vi "Export Configuration.vi"(8 "error in":errorcluster, 10 "configuration file path":path, 11 "data sharing framework custom device":T1 format="%.0x") -> (0 "error out":errorcluster, 2 "actual configuration file path":path, 3 "data sharing framework custom device":T1 format="%.0x")   [LabVIEW 2017, in "Data Sharing Framework Custom Device Scripting.lvlib"]
doc: "Creates or updates a Data Sharing Framework configuration file (.dsf) based on the custom device configuration in the system definition file."
uses:
  Data Sharing Framework Custom Device Scripting.lvlib
  <vilib>/NI Veristand/Custom Device API/Custom Device Item Ref.ctl
  Shared/DSF Shared.lvlib
  System Explorer/DSF System Explorer.lvlib
  DSF Core.lvlibp/Classes/Configuration Session/Configuration Session.lvclass
  <vilib>/NI VeriStand/Custom Device API/Custom Device API.lvlib
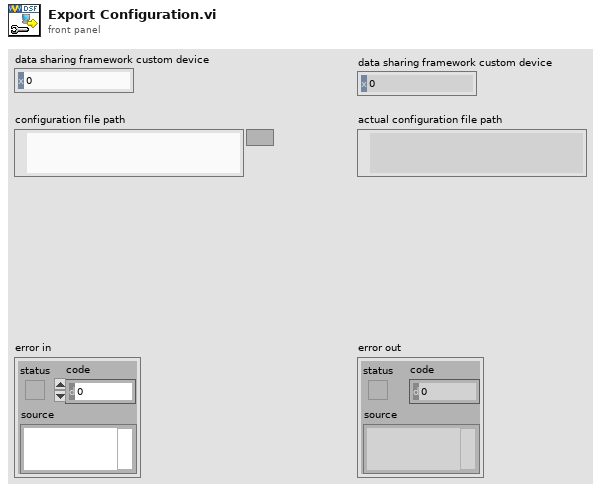
[diagram p1: front panel]
types:
  T1 = typedef "Custom Device API.lvlib/Custom Device Item Ref.ctl" = u64
  T2 = enum16{"open", "replace", "create", "open or create", "replace or create", "replace or create with confirmation"}
  T3 = typedef "DSF Core.lvlibp/DSF Engine Framework Configuration.ctl" = cluster{"plugins":T4[]}
  T4 = typedef "DSF Core.lvlibp/DSF Engine Plugin Configuration.ctl" = cluster{"core":T5, "component settings":T7[], "threads":T8[]}
  T5 = typedef "DSF Core.lvlibp/Plugin Configuration.lvclass/Core Plugin Configuration.ctl" = cluster{"name":string, "components":string[], "cycle timing":T6}
  T6 = typedef "DSF Core.lvlibp/DSF Timing Info.ctl" = cluster{"priority":u64, "decimation":u64, "offset":u64}
  T7 = typedef "DSF Core.lvlibp/DSF Settings Info.ctl" = cluster{"component":string, "values":cluster{"key":string, "value":string}[]}
  T8 = typedef "DSF Core.lvlibp/DSF Engine Plugin Thread Configuration.ctl" = cluster{"core":T9, "component settings":T7[], "transfer groups":T10[]}
  T9 = typedef "DSF Core.lvlibp/Thread Configuration.lvclass/Core Thread Configuration.ctl" = cluster{"processor":i32, "priority offset":i16}
  T10 = typedef "DSF Core.lvlibp/DSF Engine Transfer Group Configuration.ctl" = cluster{"core":T11, "component settings":T7[], "transfers":T14[]}
  T11 = typedef "DSF Core.lvlibp/Group Configuration.lvclass/Core Group Configuration.ctl" = cluster{"name":string, "direction":T12, "cycle timing":T6, "timeout behavior":T13, "enable conversion":bool}
  T12 = typedef "DSF Core.lvlibp/DSF Direction.ctl" = enum8{"Tx", "Rx"}
  T13 = typedef "DSF Core.lvlibp/DSF Timeout Behavior.ctl" = enum8{"Increment Late Count", "Throw Error"}
  T14 = typedef "DSF Core.lvlibp/DSF Engine Transfer Configuration.ctl" = cluster{"core":T15, "component settings":T7[], "channels":T16[]}
  T15 = typedef "DSF Core.lvlibp/Transfer Configuration.lvclass/Core Transfer Configuration.ctl" = cluster{"name":string}
  T16 = typedef "DSF Core.lvlibp/DSF Engine Channel Configuration.ctl" = cluster{"core":T17, "component settings":T7[]}
  T17 = typedef "DSF Core.lvlibp/Channel Configuration.lvclass/Core Channel Configuration.ctl" = cluster{"name":string, "units":string, "engine data type":T18, "string data type":T18, "string offset":u64}
  T18 = typedef "DSF Core.lvlibp/DSF Data Type.ctl" = enum8{"Bool", "SGL", "DBL", "I8", "I16", "I32", "I64", "U8", "U16", "U32", "U64"}
  T19 = typedef "DSF Core.lvlibp/DSF Version Info.ctl" = cluster{"major":u32, "minor":u32, "fix":u32, "build":string}
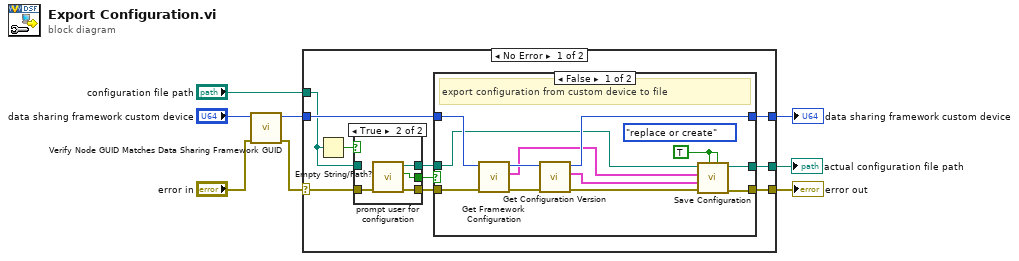
[diagram p0: block diagram]
diagram:
  n1 = call "Verify Node GUID Matches Data Sharing Framework GUID.vi"("error in"="error in", "data sharing framework custom device in"="data sharing framework custom device") -> ("error out"=w1:errorcluster, "data sharing framework custom device out"=w3:T1)  [unwired: 8 in]
  n2 = case shown="No Error" w1 {
    selector: w1 -> [w15 w42]
    tunnel: [w17 w42] -> w8
    tunnel: w3 -> [w18 w41]
    tunnel: "configuration file path" -> [w11 _]
    tunnel: [w16 w41] -> w6
    tunnel: [w9 _] -> w5
    frame No Error {
      n3 = Empty String/Path?(string/path=w11) -> (empty?=w12:bool)
      n4 = case shown="True" w12 {
        selector: w12 -> [w19 _]
        tunnel: w15 -> [w21 w25]
        tunnel: [w21 w24] -> w14
        tunnel: [w19 w23] -> w13
        tunnel: [w20 w22] -> w10
        tunnel: w11 -> [w20 _]
        frame False {
        }
        frame True {
          n5 = call "prompt user for configuration.vi"("error in (no error)"=w25) -> ("error out"=w24:errorcluster, "cancelled"=w23:bool, "selected path"=w22:path)  [unwired: 8 in]
        }
      }
      n6 = case shown="False" w13 {
        tunnel: w18 -> [w37 w40]
        tunnel: w14 -> [w34 w38]
        tunnel: [w28 w38] -> w17
        tunnel: [w35 w40] -> w16
        tunnel: w10 -> [w31 w39]
        tunnel: [w26 w39] -> w9
        frame False {
          w27 = TRUE ("create file if necessary (T)")
          (unwired) T2."replace or create" ("operation")
          # "export configuration from custom device to file"
          n7 = call "Get Framework Configuration.vi"("error in (no error)"=w34, "Item Ref in"=w37) -> ("error out"=w33:errorcluster, "framework configuration"=w29:T3, "Item Ref out"=w36:T1)  [unwired: 7 in]
          n8 = call "Get Configuration Version.vi"("error in (no error)"=w33, "Item Ref in"=w36) -> ("error out"=w32:errorcluster, "version"=w30:T19, "Item Ref out"=w35:T1)  [unwired: 7 in]
          n9 = call "Save Configuration.vi"("replace if found? (T)"=w27, "create file if necessary (T)"=w27, "error in (no error)"=w32, "version (no change)"=w30, "framework configuration"=w29, "configuration file path"=w31) -> ("error out"=w28:errorcluster, "configuration file path dup"=w26:path)  [unwired: 2 in, 2 out]
        }
        frame True {
          # "operation canceled"
        }
      }
    }
    frame Error {
    }
  }
  "data sharing framework custom device" <- w6
  "error out" <- w8
  "actual configuration file path" <- w5
